vi "SetInterfaceConfiguration.vi"(8 "ErrorIn":errorcluster, 9 "StartupConfiguration":string, 11 "IApplicationStructure":refnum<class "IApplicationConfiguration.lvclass">) -> (0 "ErrorOut":errorcluster)   [LabVIEW 2021, in "Application.lvclass"]
uses:
  Application.lvclass
  Interface_TAF_IApplicationConfiguration/IApplicationConfiguration/IApplicationConfiguration.lvclass
  852a6f4c-b1b2-4b32-b291-ab7573b75c36.vi
  <vilib>/TriekselSoft/TracerLibrary/TracerLibrary/Tracer/protected/SendMessage.vi
  <vilib>/TriekselSoft/TracerLibrary/TracerLibrary/Tracer/protected/Timestamp.vi
  852a6f4c-b1b2-4b32-b291-ab7573b75c36.vi/f75db090-0877-4668-94fb-75c2140b1617.vi
  <vilib>/TriekselSoft/TracerLibrary/TracerLibrary/Tracer/Tracer_Level-Debug.vi
  <vilib>/JDP Science/JSONtext/Variant to JSON Text.vi
  <vilib>/TriekselSoft/TracerLibrary/TracerLibrary/Tracer/protected/Tracer_ClassAttributes.vi
  <vilib>/JDP Science/JSONtext/LVClass Serializer/JSONtext LVClass Serializer.lvclass
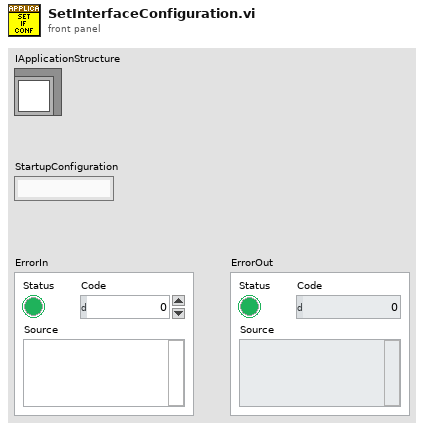
[diagram p1: front panel]
types:
  T1 = cluster{"AppConfigName":string, "class name":string}
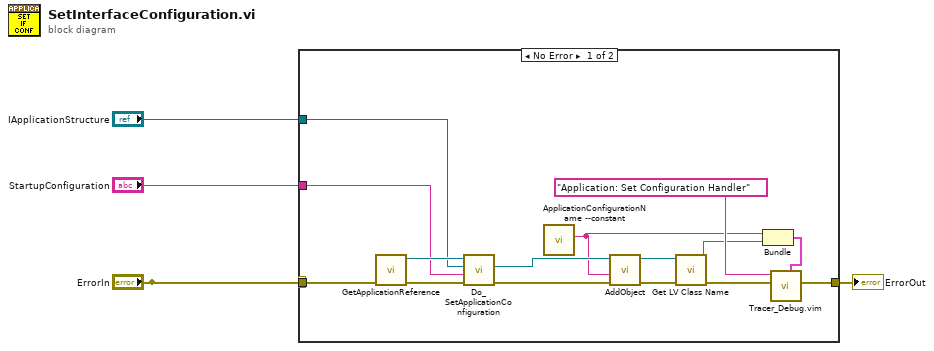
[diagram p0: block diagram]
diagram:
  n1 = case shown="No Error" "ErrorIn" {
    selector: "ErrorIn" -> [w19 w20]
    tunnel: [w16 w20] -> w4
    tunnel: "ErrorIn" -> [_ _]
    tunnel: "IApplicationStructure" -> [w11 _]
    tunnel: "StartupConfiguration" -> [w6 _]
    frame No Error {
      n2 = call "GetApplicationReference.vi"("ErrorIn"=w19) -> ("ErrorOut"=w18:errorcluster, "ApplicationOut"=w13:refnum<class "Application.lvclass">)  [unwired: 9 in]
      n3 = call-dynamic "Do_SetApplicationConfiguration.vi"("ErrorIn"=w18, "StartupConfiguration"=w6, "ConfigSource"=w11, "ApplicationIn"=w13) -> ("ErrorOut"=w17:errorcluster, "ConfigSourceOut"=w12:refnum<class "IApplicationConfiguration.lvclass">)  [unwired: 5 in, 1 out]
      n4 = call "ApplicationConfigurationName --constant.vi"() -> ("AppConfigName"=w9:string)  [unwired: 10 in, 1 out]
      n5 = call "AddObject.vi"("ErrorIn"=w17, "OjbectName"=w9, "Object2Add"=w12) -> ("ErrorOut"=w15:errorcluster, "ObjectOut"=w8:refnum<class "IApplicationConfiguration.lvclass">)  [unwired: 7 in]
      n6 = call <vilib>:"Get LV Class Name.vi"("error in (no error)"=w15, "object"=w8) -> ("error out"=w14:errorcluster, "class name"=w7:string)  [unwired: 8 in]
      n7 = Bundle("AppConfigName"=w9, "class name"=w7) -> (w5:T1)  [unwired: 1 in]
      n8 = call "Tracer_Debug.vim"("Data"=w5, "Error In"=w14, "Text"="Application: Set Configuration Handler") -> ("Error Out"=w16:errorcluster)  [unwired: 8 in]
    }
    frame Error {
    }
  }
  "ErrorOut" <- w4
